vi "250310_Nikon_Control.vi"() -> ()   [LabVIEW 2025]
doc: "This simple VI control few elements of a Nikon Ti2 microscope.\nAny kind of supplementary element can be controlled with a new event type (flurorescence cube turret for example)"
uses:
  SubVIS/Presets.ctl
panel:
  in  "Presets":T1=2 items=["1- Bino - Brightfield"=1, "2- Bino - Fluo"=2, "3- Right - Brightfield"=3, "4- Right - Fluo"=4, "5- Left"=5]
  in  "Cluster commandes":T2={"Dia lamp"=TRUE, "Dia lamp intensity"=1689.1304347826087, "Objective"=2, "Light path"=2, "Z pos (µm)"=335593, "Filter wheel 2"=2, "Filter wheel 1"=2, "Shutter 2"=TRUE, "Shutter 1"=TRUE} {"Filter wheel 1" items=["1"=1, "2"=2, "3"=3, "4"=4, "5"=5, "6"=6]; "Filter wheel 2" items=["1"=1, "2"=2, "3"=3, "4"=4, "5"=5, "6"=6]; "Z pos (µm)" min=0 max=990000 step=100 scale=0.0..990000.0; "Light path" items=["1- Eyepiece"=1, "2- Right"=2, "3- Left + Eyepiece"=3, "4- Left"=4]; "Objective" items=["1- PLAN APO 100X 1,45 Oil"=1, "2- Empty"=2, "3- Empty"=3, "4- Empty"=4, "5- Empty"=5, "6- Empty"=6]; "Dia lamp intensity" scale=0.0..2100.0}
  out "Cluster µscope":T3
  in  "stop":bool
  in  "NikonTi2AxLib.INikonTi2AxMicroscope":refnum<k7>
  out "error out":errorcluster={"status"=TRUE, "code"=-9, "source"="Exception occured in Nikon.Ti2.Microscope.1: Failed in 231026_NikonTi2_Indicators_v2.vi"} caption="sortie d'erreur"
  in  "error in":errorcluster caption="entrée d'erreur"
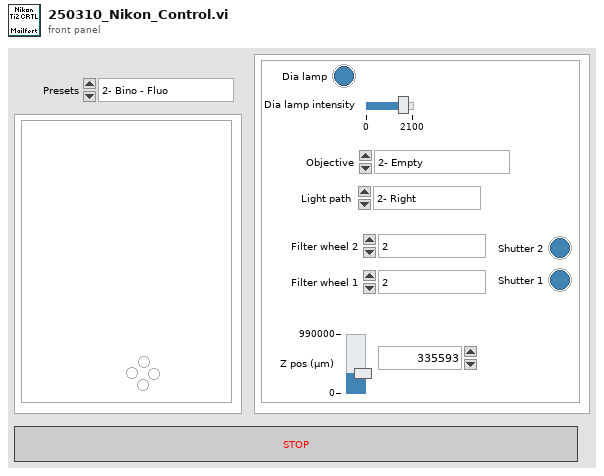
[diagram p1: front panel]
types:
  T1 = typedef "Presets.ctl" = u8
  T2 = cluster{"Dia lamp":bool, "Dia lamp intensity":dbl, "Objective":i32, "Light path":u32, "Z pos (µm)":i32, "Filter wheel 2":u32, "Filter wheel 1":u32, "Shutter 2":bool, "Shutter 1":bool}
  T3 = cluster{"Eyepiece":bool, "Right":bool, "Left + Eyepiece":bool, "Left":bool}
  T4 = cluster{"iNOSEPIECE":i32, "iLIGHTPATH":i32, "iDIA_LAMP_Switch":i32, "iDIA_LAMP_Pos":i32, "iZPOSITION":i32, "iPFS_SWITCH":i32, "iPFS_STATUS":i32, "iPFS_OFFSET":i32, "iTURRET2POS":i32, "Turret2SHUTTER":i32, "iTURRET1POS":i32, "Turret1SHUTTER":i32}
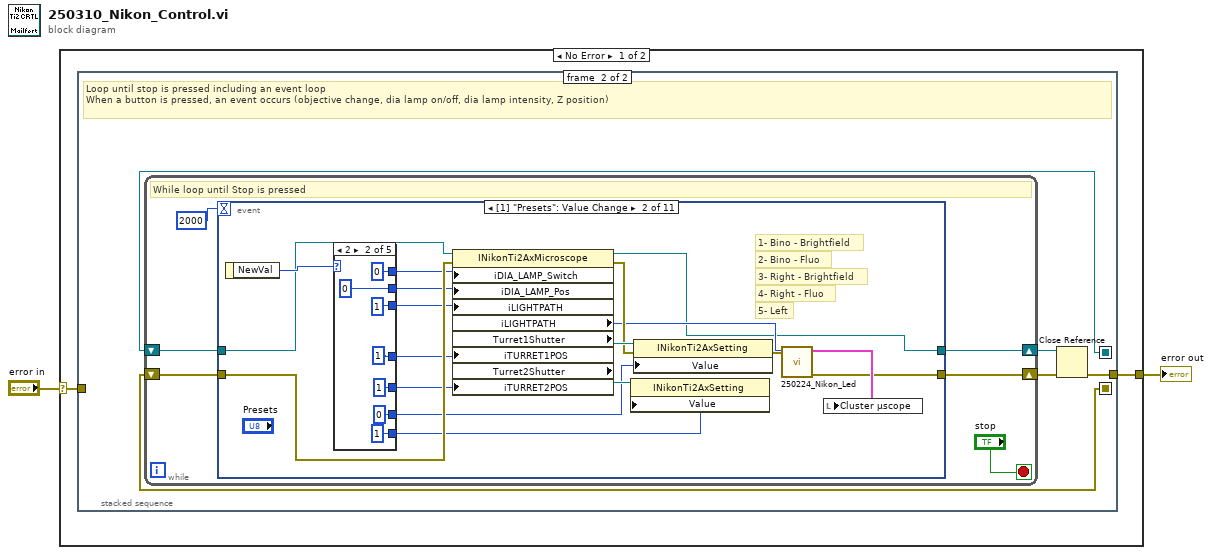
[diagram p0: block diagram]
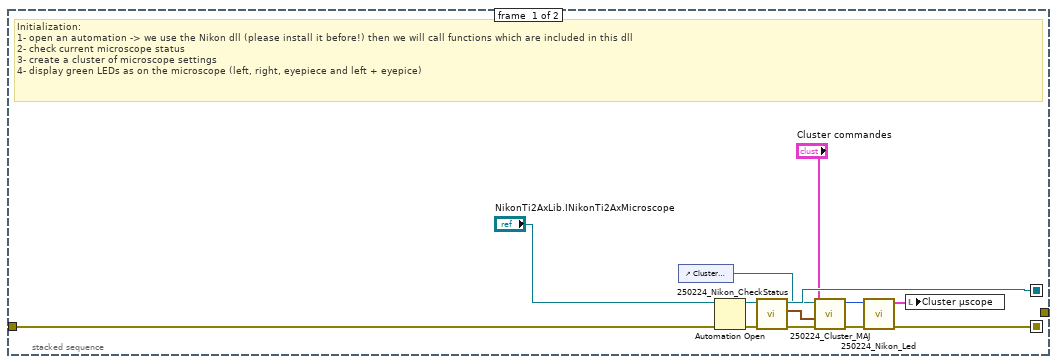
[diagram p2: hidden frame]
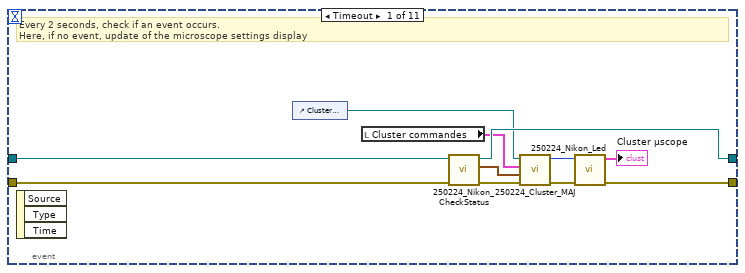
[diagram p3: hidden frame]
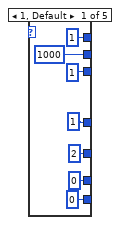
[diagram p4: hidden frame]
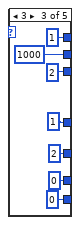
[diagram p5: hidden frame]
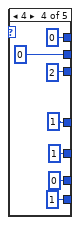
[diagram p6: hidden frame]
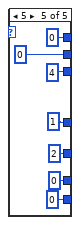
[diagram p7: hidden frame]
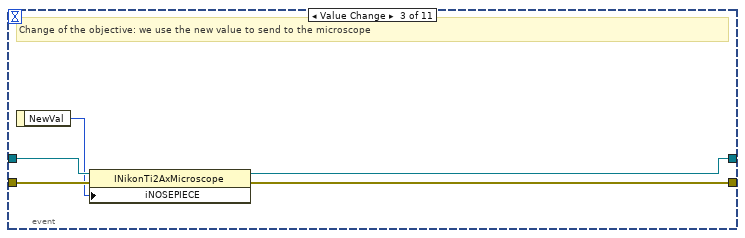
[diagram p8: hidden frame]
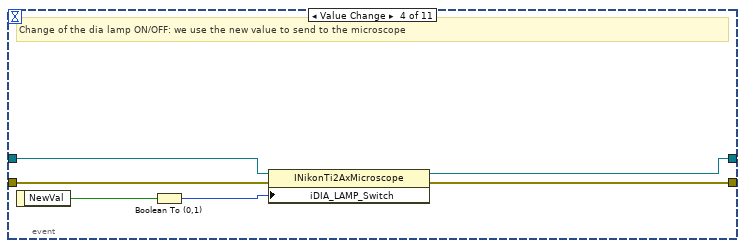
[diagram p9: hidden frame]
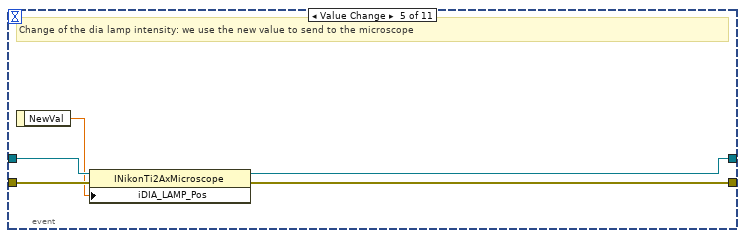
[diagram p10: hidden frame]
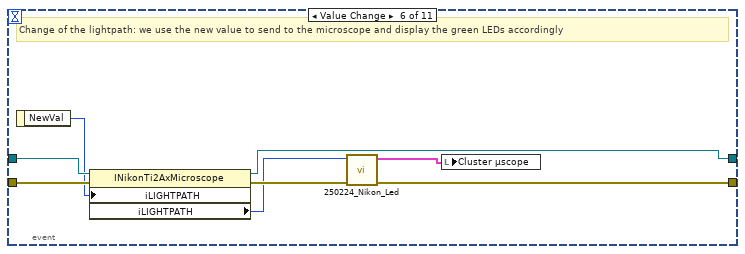
[diagram p11: hidden frame]
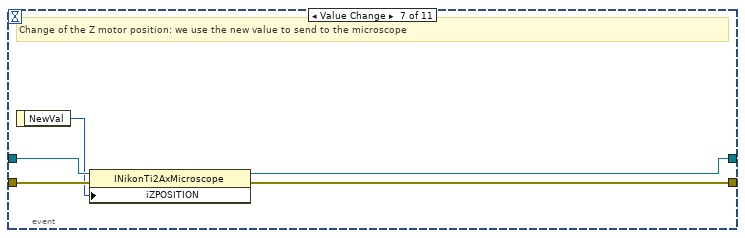
[diagram p12: hidden frame]
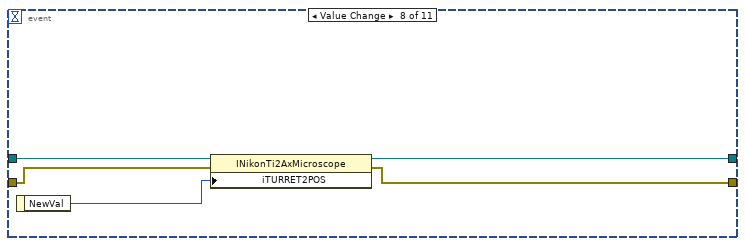
[diagram p13: hidden frame]
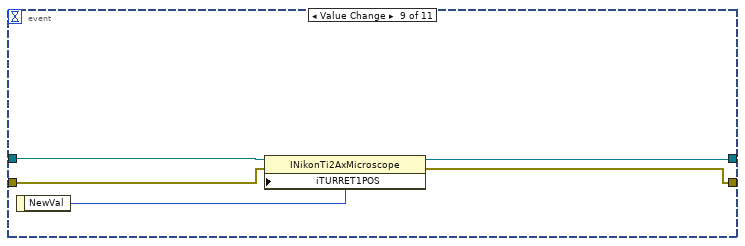
[diagram p14: hidden frame]
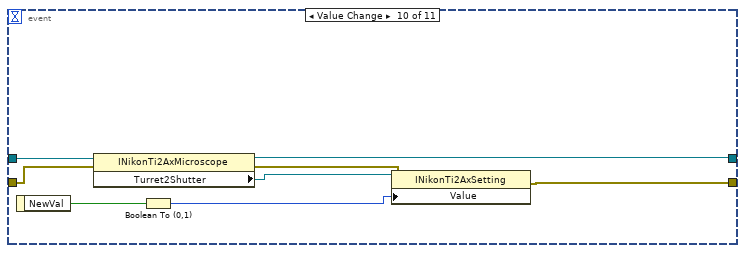
[diagram p15: hidden frame]
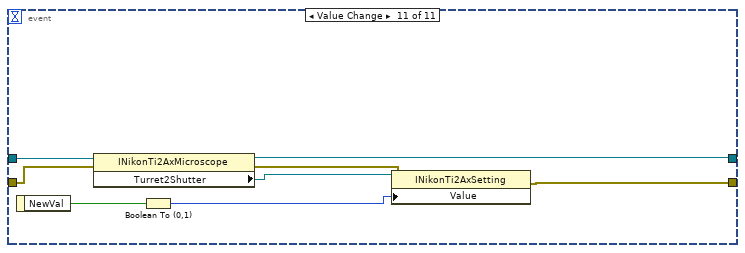
[diagram p16: hidden frame]
diagram:
  n1 = case shown="No Error" "error in" {
    selector: "error in" -> [w4 w148]
    tunnel: [w3 w148] -> w1
    frame No Error {
      n2 = stacked-sequence {
        seq-local: [w13 _] -> [_ w22]
        seq-local: [w7 _] -> [_ w18]
        tunnel: w4 -> [w14 _]
        tunnel: [_ w19] -> w3
        frame #0 {
          # "Initialization:\n1- open an automation -> we use the Nikon dll (please install it before!) then we will call functions which are included in this dll\n2- check current microscope status\n3- create a cluster of microscope settings\n4- display green LEDs as on the microscope (left, right, eyepiece and left + eyepice)"
          n3 = control-ref of="Cluster commandes"() -> (w6:refnum<vi>)
          n4 = Automation Open(error in (no error)=w14, Automation Refnum="NikonTi2AxLib.INikonTi2AxMicroscope") -> (Automation Refnum=w16:refnum<k7>, error out=w15:errorcluster)  [unwired: 2 in]
          n5 = call "250224_Nikon_CheckStatus.vi"("error in"=w15, "NikonTi2AxLib.INikonTi2AxMicroscope"=w16) -> ("error out"=w9:errorcluster, "Nikon status cluster"=w12:T4, "reference out"=w13:refnum<k7>)  [unwired: 7 in]
          n6 = call "250224_Cluster_MAJ.vi"("error in (no error)"=w9, "Nikon status cluster"=w12, 10:"Cluster commandes"="Cluster commandes", 11:"Cluster commandes"=w6) -> ("error out"=w8:errorcluster, "iLIGHTPATH"=w10:i32)  [unwired: 6 in]
          n7 = call "250224_Nikon_Led.vi"("error in"=w8, "Light path"=w10) -> ("error out"=w7:errorcluster, "Cluster µscope"=w11:T3)  [unwired: 8 in]
          n8 = local write "Cluster µscope"(w11) -> ()
        }
        frame #1 {
          # "Loop until stop is pressed including an event loop\nWhen a button is pressed, an event occurs (objective change, dia lamp on/off, dia lamp intensity, Z position)"
          n9 = while {
            shift-right: [w23] -> w20
            shift-left: w18 -> [w28]
            shift-right: [w24] -> w21
            shift-left: w22 -> [w25]
            stop <- "stop" stop-if-true
            # "While loop until Stop is pressed"
            n10 = event shown="[1] \"Presets\": Value Change" {
              selector: _ -> [_ _ _ _ _ _ _ _ _ _ _]
              dyn-events: _ -> [_ _ _ _ _ _ _ _ _ _ _]
              timeout: 2000 -> [_ _ _ _ _ _ _ _ _ _ _]
              tunnel: [w36 w56 w94 w100 w105 w113 w120 w123 w127 w134 w142] -> w23
              tunnel: w28 -> [w39 w51 w96 w102 w107 w114 w118 w124 w130 w139 w147]
              tunnel: w25 -> [w38 w52 w97 w103 w108 w115 w119 w126 w131 w138 w146]
              tunnel: [w37 w40 w95 w101 w106 w116 w121 w122 w128 w135 w143] -> w24
              event Timeout {
                # "Every 2 seconds, check if an event occurs.\nHere, if no event, update of the microscope settings display"
                n11 = event-data() -> ()  [unwired: 1 in, 3 out]
                n12 = control-ref of="Cluster commandes"() -> (w29:refnum<vi>)
                n13 = local read "Cluster commandes"() -> (w30:T2)
                n14 = call "250224_Nikon_CheckStatus.vi"("error in"=w39, "NikonTi2AxLib.INikonTi2AxMicroscope"=w38) -> ("error out"=w33:errorcluster, "Nikon status cluster"=w34:T4, "reference out"=w37:refnum<k7>)  [unwired: 7 in]
                n15 = call "250224_Cluster_MAJ.vi"("error in (no error)"=w33, "Nikon status cluster"=w34, 10:"Cluster commandes"=w30, 11:"Cluster commandes"=w29) -> ("error out"=w32:errorcluster, "iLIGHTPATH"=w31:i32)  [unwired: 6 in]
                n16 = call "250224_Nikon_Led.vi"("error in"=w32, "Light path"=w31) -> ("error out"=w36:errorcluster, "Cluster µscope"=→"Cluster µscope":T3)  [unwired: 8 in]
              }
              event Value Change {
                # "1- Bino - Brightfield"
                # "5- Left"
                # "4- Right - Fluo"
                # "3- Right - Brightfield"
                # "2- Bino - Fluo"
                n17 = event-data() -> ("NewVal"=w55:T1)  [unwired: 1 in]
                n18 = case shown="2" w55 {
                  tunnel: [1 0 1 0 0] -> w47
                  tunnel: [1000 0 1000 0 0] -> w46
                  tunnel: [1 ("iLIGHTPATH") 1 ("iLIGHTPATH") 2 ("iLIGHTPATH") 2 ("iLIGHTPATH") 4 ("iLIGHTPATH")] -> w45
                  tunnel: [1 ("iLIGHTPATH") 1 ("iLIGHTPATH") 1 ("iLIGHTPATH") 1 ("iLIGHTPATH") 1 ("iLIGHTPATH")] -> w44
                  tunnel: [2 ("iLIGHTPATH") 1 ("iLIGHTPATH") 2 ("iLIGHTPATH") 1 ("iLIGHTPATH") 2 ("iLIGHTPATH")] -> w43
                  tunnel: [0 ("iLIGHTPATH") 0 ("iLIGHTPATH") 0 ("iLIGHTPATH") 0 ("iLIGHTPATH") 0 ("iLIGHTPATH")] -> w42
                  tunnel: [0 ("iLIGHTPATH") 1 ("iLIGHTPATH") 0 ("iLIGHTPATH") 1 ("iLIGHTPATH") 0 ("iLIGHTPATH")] -> w41
                  frame 1, Default {
                  }
                  frame 2 {
                  }
                  frame 3 {
                  }
                  frame 4 {
                  }
                  frame 5 {
                  }
                }
                n19 = property class="INikonTi2AxMicroscope"(reference=w52, error in=w51, "iDIA_LAMP_Switch"=w47, "iDIA_LAMP_Pos"=w46, "iLIGHTPATH"=w45, "iTURRET1POS"=w44, "iTURRET2POS"=w43) -> (reference out=w40:refnum<k7>, error out=w50:errorcluster, "iLIGHTPATH"=w48:i32, "Turret1Shutter"=w54:refnum<k7>, "Turret2Shutter"=w53:refnum<k7>)
                n20 = property class="INikonTi2AxSetting"(reference=w53, "Value"=w41) -> ()  [unwired: 1 in, 2 out]
                n21 = property class="INikonTi2AxSetting"(reference=w54, error in=w50, "Value"=w42) -> (error out=w49:errorcluster)  [unwired: 1 out]
                n22 = call "250224_Nikon_Led.vi"("error in"=w49, "Light path"=w48) -> ("error out"=w56:errorcluster, "Cluster µscope"=w57:T3)  [unwired: 8 in]
                n23 = local write "Cluster µscope"(w57) -> ()
              }
              event "Cluster commandes.Objective": Value Change {
                # "Change of the objective: we use the new value to send to the microscope"
                n24 = event-data() -> ("NewVal"=w93:i32)  [unwired: 1 in]
                n25 = property class="INikonTi2AxMicroscope"(reference=w97, error in=w96, "iNOSEPIECE"=w93) -> (reference out=w95:refnum<k7>, error out=w94:errorcluster)
              }
              event "Cluster commandes.Dia lamp": Value Change {
                # "Change of the dia lamp ON/OFF: we use the new value to send to the microscope"
                n26 = event-data() -> ("NewVal"=w99:bool)  [unwired: 1 in]
                n27 = Boolean To (0,1)(Boolean=w99) -> (0, 1=w98:i16)
                n28 = property class="INikonTi2AxMicroscope"(reference=w103, error in=w102, "iDIA_LAMP_Switch"=w98) -> (reference out=w101:refnum<k7>, error out=w100:errorcluster)
              }
              event "Cluster commandes.Dia lamp intensity": Value Change {
                # "Change of the dia lamp intensity: we use the new value to send to the microscope"
                n29 = event-data() -> ("NewVal"=w104:dbl)  [unwired: 1 in]
                n30 = property class="INikonTi2AxMicroscope"(reference=w108, error in=w107, "iDIA_LAMP_Pos"=w104) -> (reference out=w106:refnum<k7>, error out=w105:errorcluster)
              }
              event "Cluster commandes.Light path": Value Change {
                # "Change of the lightpath: we use the new value to send to the microscope and display the green LEDs accordingly"
                n31 = event-data() -> ("NewVal"=w110:u32)  [unwired: 1 in]
                n32 = property class="INikonTi2AxMicroscope"(reference=w115, error in=w114, "iLIGHTPATH"=w110) -> (reference out=w116:refnum<k7>, error out=w112:errorcluster, "iLIGHTPATH"=w111:i32)
                n33 = call "250224_Nikon_Led.vi"("error in"=w112, "Light path"=w111) -> ("error out"=w113:errorcluster, "Cluster µscope"=w109:T3)  [unwired: 8 in]
                n34 = local write "Cluster µscope"(w109) -> ()
              }
              event "Cluster commandes.Z pos (µm)": Value Change {
                # "Change of the Z motor position: we use the new value to send to the microscope"
                n35 = event-data() -> ("NewVal"=w117:i32)  [unwired: 1 in]
                n36 = property class="INikonTi2AxMicroscope"(reference=w119, error in=w118, "iZPOSITION"=w117) -> (reference out=w121:refnum<k7>, error out=w120:errorcluster)
              }
              event "Cluster commandes.Filter wheel 2": Value Change {
                n37 = event-data() -> ("NewVal"=w125:u32)  [unwired: 1 in]
                n38 = property class="INikonTi2AxMicroscope"(reference=w126, error in=w124, "iTURRET2POS"=w125) -> (reference out=w122:refnum<k7>, error out=w123:errorcluster)
              }
              event "Cluster commandes.Filter wheel 1": Value Change {
                n39 = event-data() -> ("NewVal"=w129:u32)  [unwired: 1 in]
                n40 = property class="INikonTi2AxMicroscope"(reference=w131, error in=w130, "iTURRET1POS"=w129) -> (reference out=w128:refnum<k7>, error out=w127:errorcluster)
              }
              event "Cluster commandes.Shutter 2": Value Change {
                n41 = event-data() -> ("NewVal"=w133:bool)  [unwired: 1 in]
                n42 = property class="INikonTi2AxMicroscope"(reference=w138, error in=w139) -> (reference out=w135:refnum<k7>, error out=w136:errorcluster, "Turret2Shutter"=w137:refnum<k7>)
                n43 = Boolean To (0,1)(Boolean=w133) -> (0, 1=w132:i16)
                n44 = property class="INikonTi2AxSetting"(reference=w137, error in=w136, "Value"=w132) -> (error out=w134:errorcluster)  [unwired: 1 out]
              }
              event "Cluster commandes.Shutter 1": Value Change {
                n45 = event-data() -> ("NewVal"=w141:bool)  [unwired: 1 in]
                n46 = property class="INikonTi2AxMicroscope"(reference=w146, error in=w147) -> (reference out=w143:refnum<k7>, error out=w144:errorcluster, "Turret2Shutter"=w145:refnum<k7>)
                n47 = Boolean To (0,1)(Boolean=w141) -> (0, 1=w140:i16)
                n48 = property class="INikonTi2AxSetting"(reference=w145, error in=w144, "Value"=w140) -> (error out=w142:errorcluster)  [unwired: 1 out]
              }
            }
          }
          n49 = Close Reference(reference=w21, error in (no error)=w20) -> (error out=w19:errorcluster)
        }
      }
    }
    frame Error {
    }
  }
  "error out" <- w1
